vi "Set Sub Panel Prods.vi"(8 "error in (no error)":errorcluster, 10 "Sub Panel Prods":refnum<vi>, 11 "Coca Actors in":refnum<class "Coca Actors.lvclass">) -> (0 "error out":errorcluster, 3 "Coca Actors out":refnum<class "Coca Actors.lvclass">)   [LabVIEW 2020, in "Coca Actors.lvlib" / "Coca Actors.lvclass"]
uses:
  Coca Actors.lvclass
  Coca Actors.lvclass/Coca Actors.ctl
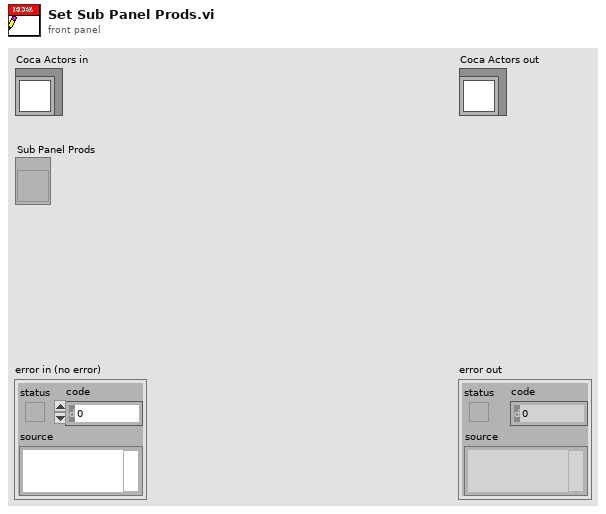
[diagram p1: front panel]
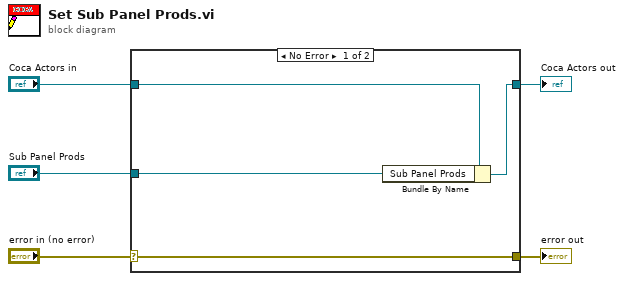
[diagram p0: block diagram]
diagram:
  n1 = case shown="No Error" "error in (no error)" {
    selector: "error in (no error)" -> [w9 w10]
    tunnel: [w9 w10] -> w4
    tunnel: [w7 w11] -> w2
    tunnel: "Coca Actors in" -> [w8 w11]
    tunnel: "Sub Panel Prods" -> [w6 _]
    frame No Error {
      n2 = Bundle By Name(cluster=w8, "Sub Panel Prods"=w6) -> (w7:refnum<class "Coca Actors.lvclass">)
    }
    frame Error {
    }
  }
  "error out" <- w4
  "Coca Actors out" <- w2
